vi "FacadeResizable2DArray(U16).vi"(0 "Data In":T4, 2 "Display State In":T2, 3 "Container State":T3) -> (6 "Data Out":T4, 7 "Display State Out":T2, 8 "Action":T1)   [LabVIEW 2011, in "Resizable2DArray(U16).xctl"]
uses:
  <vilib>/_probes/SAPHIR/ViBox - Probes/Resizable2DArray/Resizable2DArray(U16)/Resizable2DArray(U16).xctl
  <vilib>/_probes/SAPHIR/ViBox - Probes/Resizable2DArray/Resizable2DArray(U16)/DataResizable2DArray(U16).ctl
  <vilib>/_xctls/Container State.ctl
  <vilib>/_probes/SAPHIR/ViBox - Probes/Resizable2DArray/Resizable2DArray(U16)/StateResizable2DArray(U16).ctl
  <vilib>/_xctls/Action.ctl
  <vilib>/_xctls/XControlSupport.lvlib
panel:
  in  "Format":string caption="Format :"
  out "Numeric":u16
  out "[U16]":u16[][](array[numeric])
  # "Display Options"
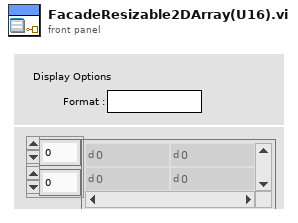
[diagram p1: front panel]
types:
  T1 = typedef "XControlSupport.lvlib/Action.ctl" = cluster{"Data Changed?":bool, "State Changed?":bool, "Action Name":string}
  T2 = typedef "Resizable2DArray(U16).xctl/StateResizable2DArray(U16).ctl" = cluster{"Height":u32, "Width":u32, "TextWidth":u32}
  T3 = typedef "XControlSupport.lvlib/Container State.ctl" = cluster{"Indicator?":bool, "Run Mode?":bool, " Refnum":refnum<vi>}
  T4 = typedef "Resizable2DArray(U16).xctl/DataResizable2DArray(U16).ctl" = u16[][]
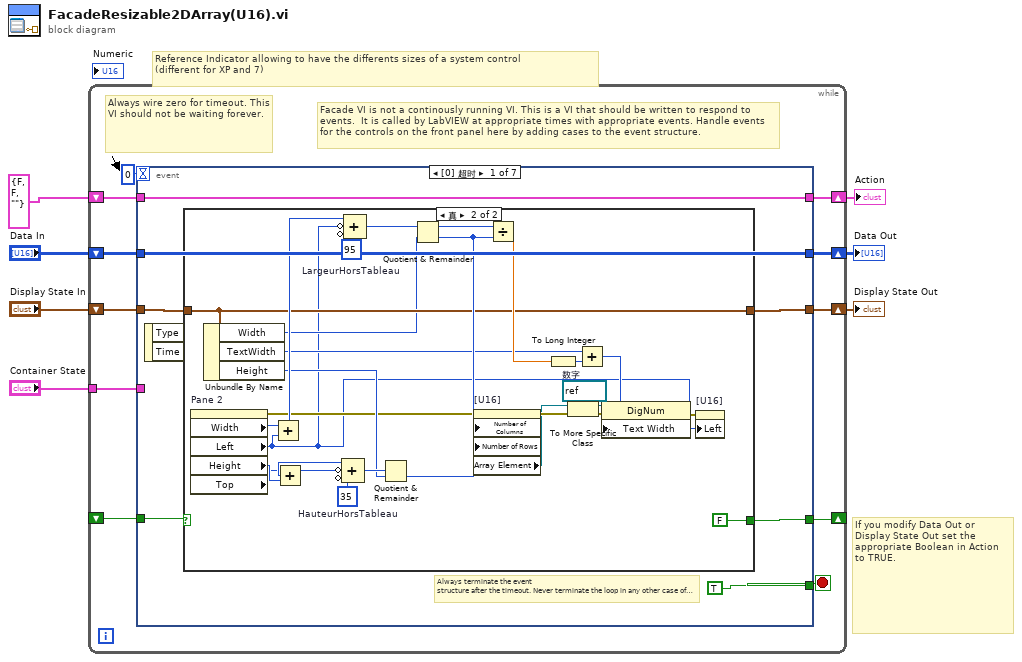
[diagram p0: block diagram]
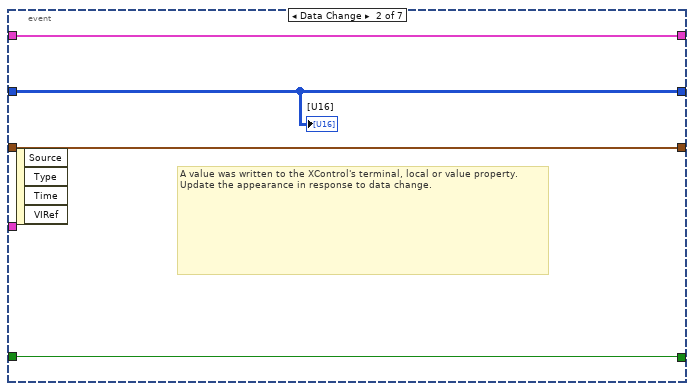
[diagram p3: hidden frame]
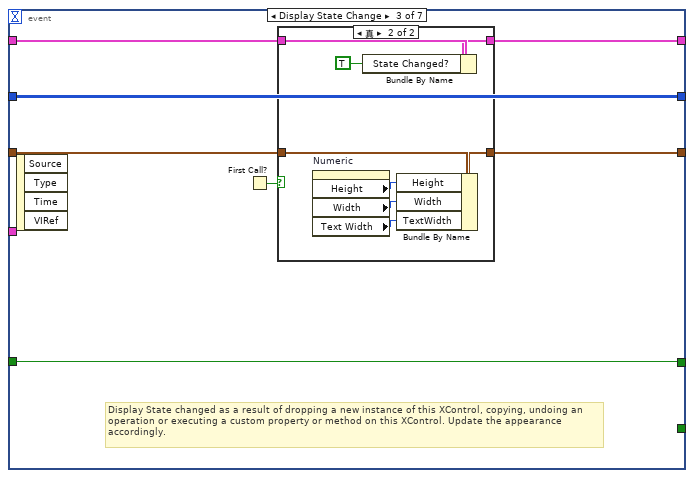
[diagram p4: hidden frame]
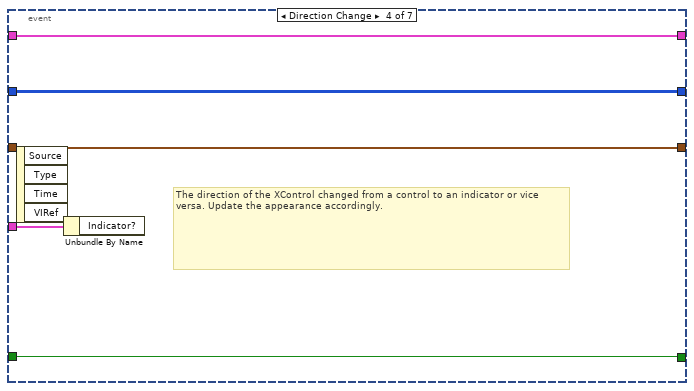
[diagram p6: hidden frame]
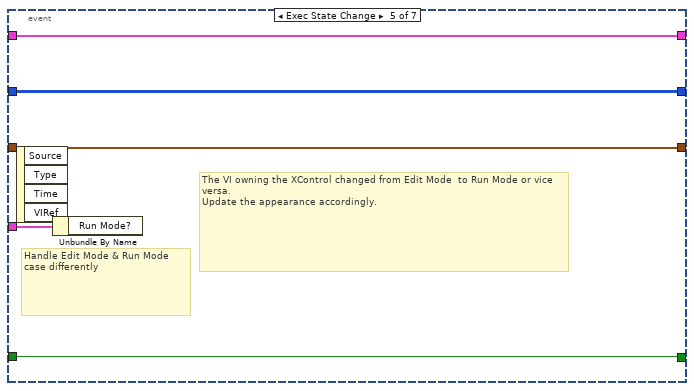
[diagram p7: hidden frame]
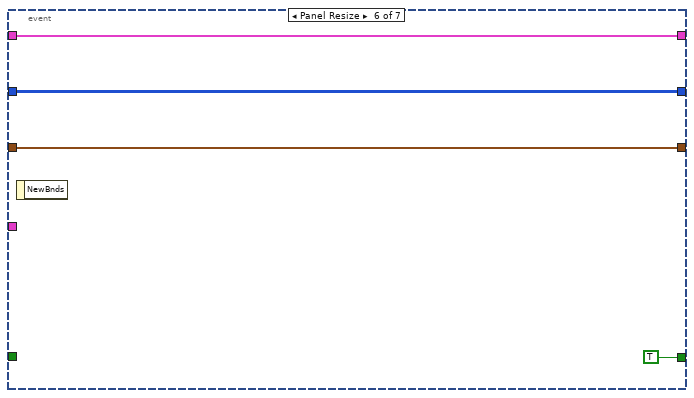
[diagram p8: hidden frame]
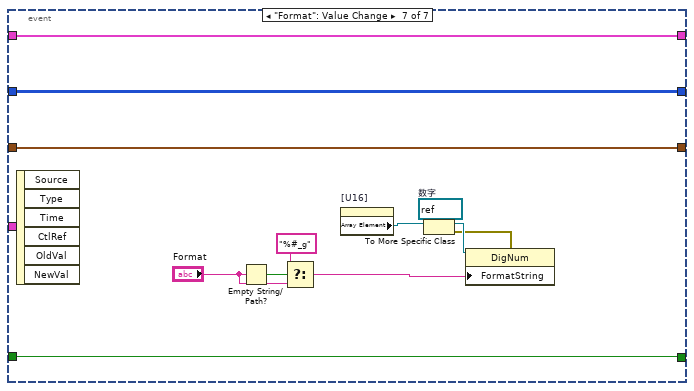
[diagram p9: hidden frame]
diagram:
  # "Reference Indicator allowing to have the differents sizes of a system control\n(different for XP and 7)"
  # "If you modify Data Out or\nDisplay State Out set the\nappropriate Boolean in Action\nto TRUE."
  n1 = while {
    shift-right: [w17] -> w5
    shift-left: "Display State In" -> [w18]
    tunnel: "Container State" -> [w14]
    shift-right: [w12] -> w7
    shift-left: "Data In" -> [w13]
    shift-right: [w10] -> w3
    shift-left: T1 {"Data Changed?"=FALSE, "State Changed?"=FALSE, "Action Name"=""} ("Action") -> [w11]
    shift-right: [w8] -> _
    shift-left: _ -> [w9]
    stop <- w16 stop-if-true
    # "Facade VI is not a continously running VI. This is a VI that should be written to respond to events.  It is called by LabVIEW at appropriate times with appropriate events. Handle events for the controls on the front panel here by adding cases to the event structure."
    # "Always wire zero for timeout. This\nVI should not be waiting forever."
    n2 = event shown="[0] 超时" {
      selector: _ -> [_ _ _ _ _ _ _]
      dyn-events: _ -> [_ _ _ _ _ _ _]
      timeout: 0 -> [_ _ _ _ _ _ _]
      tunnel: w18 -> [w21 w59 w64 w80 w85 w88 w99]
      tunnel: [w20 w59 w63 w80 w85 w88 w99] -> w17
      tunnel: [TRUE _ _ _ _ _ _] -> w16
      tunnel: w14 -> [_ _ _ w81 w86 _ _]
      tunnel: w13 -> [w23 w57 w66 w79 w84 w90 w100]
      tunnel: [w23 w57 w66 w79 w84 w90 w100] -> w12
      tunnel: [w24 w58 w61 w78 w83 w89 w101] -> w10
      tunnel: w11 -> [w24 w58 w62 w78 w83 w89 w101]
      tunnel: w9 -> [w22 w56 w65 w77 w82 _ w102]
      tunnel: [w19 w56 w65 w77 w82 TRUE w102] -> w8
      event Timeout {
        # "Always terminate the event\nstructure after the timeout. Never terminate the loop in any other case of the event structure."
        n3 = event-data() -> ()  [unwired: 3 out]
        n4 = case shown="真" w22 {
          selector: w22 -> [w27 _]
          tunnel: w21 -> [w26 w37]
          tunnel: [w26 w37] -> w20
          tunnel: [w27 FALSE] -> w19
          frame False {
          }
          frame True {
            w44 = refnum<vi> refnum  # 数字
            w42 = i16 35  # HauteurHorsTableau
            w43 = i16 95  # LargeurHorsTableau
            n5 = property on="Pane 2" class="Pane"() -> (error out=w31:errorcluster, "Width"=w32:u32, "Left"=w30:i32, "Height"=w29:u32, "Top"=w28:i32)  [unwired: 2 in, 1 out]
            n6 = Unbundle By Name(w37) -> ("Width"=w36:u32, "TextWidth"=w35:u32, "Height"=w34:u32)
            n7 = Add(x=w32, y=w30) -> (x+y=w41:u32)
            n8 = Add(x=w28, y=w29) -> (x+y=w55:u32)
            n9 = Compound Arithmetic op=ADD(w55, invert w28, invert w42) -> (w51:u32)
            n10 = Compound Arithmetic op=ADD(w41, invert w30, invert w43) -> (w47:u32)
            n11 = Quotient & Remainder(x=w51, y=w34) -> (floor(x/y)=w38:u32)  [unwired: 1 out]
            n12 = Quotient & Remainder(x=w47, y=w36) -> (x-y*floor(x/y)=w40:u32, floor(x/y)=w39:u32)
            n13 = property on="[U16]" class="Arr (严格)"(error in=w31, "Number of Columns"=w39, "Number of Rows"=w38) -> (error out=w52:errorcluster, "Array Element"=w50:refnum<vi>)  [unwired: 1 in, 1 out]
            n14 = Divide(x=w40, y=w39) -> (x/y=w48:dbl)
            n15 = To Long Integer(number=w48) -> (32bit integer=w49:i32)
            n16 = To More Specific Class(target class=w44, reference=w50, error in=w52) -> (specific class reference=w45:refnum<vi>, error out=w53:errorcluster)
            n17 = Add(x=w35, y=w49) -> (x+y=w46:u32)
            n18 = property class="DigNum"(reference=w45, error in=w53, "Text Width"=w46) -> (error out=w54:errorcluster)  [unwired: 1 out]
            n19 = property on="[U16]" class="Arr (严格)"(error in=w54, "Left"=w30) -> ()  [unwired: 1 in, 2 out]
          }
        }
      }
      event Data Change {
        # "A value was written to the XControl's terminal, local or value property.\nUpdate the appearance in response to data change."
        n20 = event-data() -> ()  [unwired: 5 out]
        "[U16]" <- w57
      }
      event Display State Change {
        # "Display State changed as a result of dropping a new instance of this XControl, copying, undoing an operation or executing a custom property or method on this XControl. Update the appearance accordingly."
        n21 = event-data() -> ()  [unwired: 5 out]
        n22 = First Call?() -> (First Call?: T/F=w60:bool)
        n23 = case shown="真" w60 {
          tunnel: w64 -> [w68 w76]
          tunnel: [w68 w75] -> w63
          tunnel: w62 -> [w67 w73]
          tunnel: [w67 w69] -> w61
          frame False {
          }
          frame True {
            n24 = property on="Numeric" class="DigNum (严格)"() -> ("Height"=w74:u32, "Width"=w71:u32, "Text Width"=w70:u32)  [unwired: 2 in, 2 out]
            n25 = Bundle By Name(cluster=w73, "State Changed?"=TRUE) -> (w69:T1)
            n26 = Bundle By Name(cluster=w76, "Height"=w74, "Width"=w71, "TextWidth"=w70) -> (w75:T2)
          }
        }
      }
      event Direction Change {
        # "The direction of the XControl changed from a control to an indicator or vice versa. Update the appearance accordingly."
        n27 = event-data() -> ()  [unwired: 5 out]
        n28 = Unbundle By Name(w81) -> ()  [unwired: 1 out]
      }
      event Exec State Change {
        # "The VI owning the XControl changed from Edit Mode  to Run Mode or vice versa.\nUpdate the appearance accordingly."
        # "Handle Edit Mode & Run Mode\ncase differently"
        n29 = event-data() -> ()  [unwired: 5 out]
        n30 = Unbundle By Name(w86) -> ()  [unwired: 1 out]
      }
      event Panel Resize {
        n31 = event-data() -> ()  [unwired: 2 out]
      }
      event "Format": Value Change {
        w98 = refnum<vi> refnum  # 数字
        n32 = event-data() -> ()  [unwired: 7 out]
        n33 = Empty String/Path?(string/path="Format") -> (empty?=w94:bool)
        n34 = Select(t="%#_g", s=w94, f="Format") -> (s? t:f=w92:string)
        n35 = property on="[U16]" class="Arr (严格)"() -> ("Array Element"=w95:refnum<vi>)  [unwired: 2 in, 2 out]
        n36 = To More Specific Class(target class=w98, reference=w95) -> (specific class reference=w97:refnum<vi>, error out=w96:errorcluster)  [unwired: 1 in]
        n37 = property class="DigNum"(reference=w97, error in=w96, "FormatString"=w92) -> ()  [unwired: 2 out]
      }
    }
  }
  "Display State Out" <- w5
  "Data Out" <- w7
  "Action" <- w3
